vi "DPCal-Find Optimal Attenuation.vi"(7 "Nominal Max SPL":dbl[](array[numeric]), 11 "error in (no error)":errorcluster) -> (8 "Attenuation (dB)":dbl[](array[numeric]), 15 "error out":errorcluster)   [LabVIEW 2020]
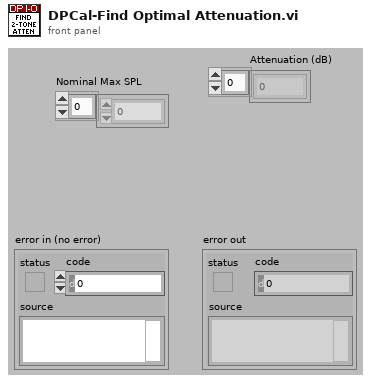
[diagram p1: front panel]
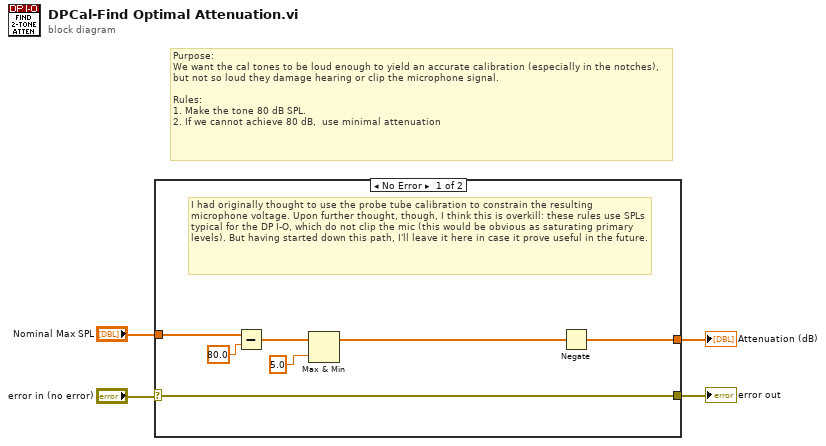
[diagram p0: block diagram]
diagram:
  # "Purpose: \nWe want the cal tones to be loud enough to yield an accurate calibration (especially in the notches), but not so loud they damage hearing or clip the microphone signal.\n\nRules: \n1. Make the tone 80 dB SPL.\n2. If we cannot achieve 80 dB,  use minimal attenuation"
  n1 = case shown="No Error" "error in (no error)" {
    selector: "error in (no error)" -> [w11 w12]
    tunnel: [w11 w12] -> w3
    tunnel: "Nominal Max SPL" -> [w10 _]
    tunnel: [w5 _] -> w1
    frame No Error {
      # "I had originally thought to use the probe tube calibration to constrain the resulting microphone voltage. Upon further thought, though, I think this is overkill: these rules use SPLs typical for the DP I-O, which do not clip the mic (this would be obvious as saturating primary levels). But having started down this path, I'll leave it here in case it prove useful in the future."
      n2 = Subtract(x=w10, y=80.0) -> (x-y=w8:dbl[])
      n3 = Max & Min(x=w8, y=5.0) -> (max(x,y)=w6:dbl[])  [unwired: 1 out]
      n4 = Negate(x=w6) -> (-x=w5:dbl[])
    }
    frame Error {
    }
  }
  "error out" <- w3
  "Attenuation (dB)" <- w1
